vi "Kreise_sortieren.vi"(11 "Circles in":T1(array[cluster])) -> (3 "Circles out":T1(array[cluster]))   [LabVIEW 2024]
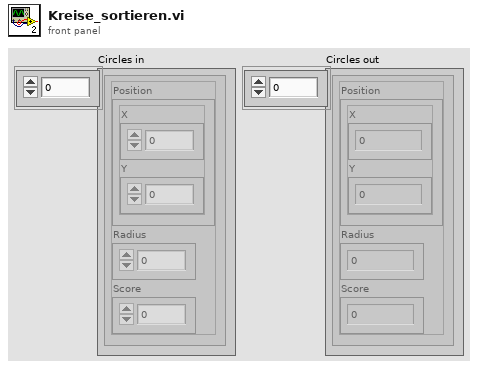
[diagram p1: front panel]
types:
  T1 = cluster{"Position":cluster{"X":sgl, "Y":sgl}, "Radius":dbl, "Score":dbl}[]
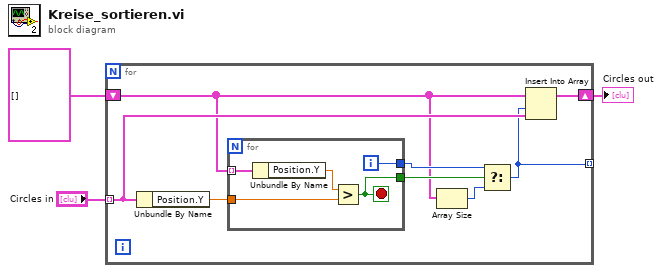
[diagram p0: block diagram]
diagram:
  n1 = for {
    tunnel: "Circles in" -> [w9] mode=indexing
    shift-right: [w11] -> w2
    shift-left: T1 [] ("Circles in") -> [w5]
    tunnel: [w6] -> _ mode=indexing
    n2 = Unbundle By Name(w9) -> ("Position.Y"=w10:sgl)
    n3 = for {
      tunnel: w5 -> [w16] mode=indexing
      tunnel: w10 -> [w14]
      tunnel: [w13] -> w7
      tunnel: [w12] -> w8
      i -> [w13]
      stop <- w12 stop-if-true
      n4 = Unbundle By Name(w16) -> ("Position.Y"=w15:sgl)
      n5 = Greater?(x=w15, y=w14) -> (0:w12:bool)
    }
    n6 = Array Size(array=w5) -> (size(s)=w4:i32)
    n7 = Select(t=w7, s=w8, f=w4) -> (s? t:f=w6:i32)
    n8 = Insert Into Array(array=w5, index=w6, new element=w9) -> (w11:T1)
  }
  "Circles out" <- w2
